vi "WLAN Rx Test Set WLAN INSTR RX.vi"(8 "error in (no error)":errorcluster, 10 "niDTS WLAN.lvlib:niDTS WLAN INSTR RX":refnum<class "niDTS WLAN INSTR RX.lvclass">, 11 "niDTS WLAN Rx Test in":refnum<class "niDTS WLAN Rx Test.lvclass">) -> (0 "error out":errorcluster, 3 "niDTS WLAN Rx Test out":refnum<class "niDTS WLAN Rx Test.lvclass">)   [LabVIEW 2015, in "niDTS WLAN.lvlib" / "niDTS WLAN Rx Test.lvclass"]
uses:
  niDTS WLAN Rx Test.lvclass
  Instrument/INSTR RX/niDTS WLAN INSTR RX.lvclass
  niDTS WLAN Rx Test.lvclass/niDTS WLAN Rx Test.ctl
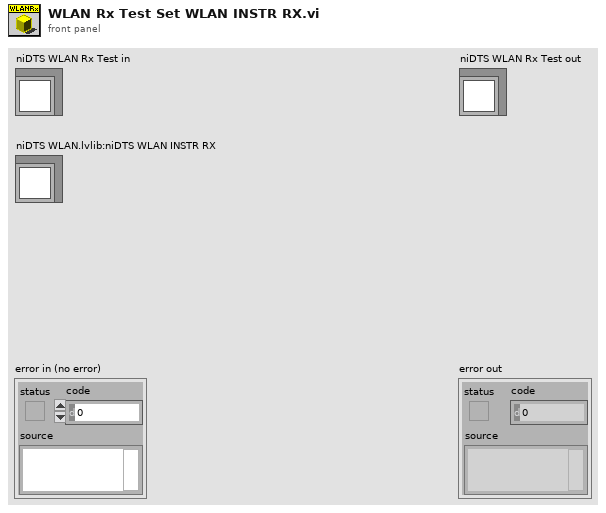
[diagram p1: front panel]
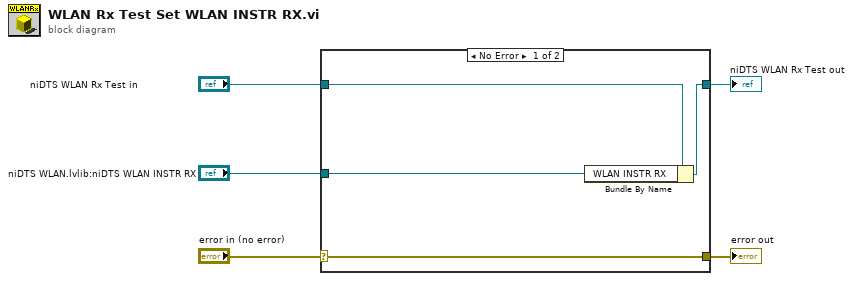
[diagram p0: block diagram]
diagram:
  n1 = case shown="No Error" "error in (no error)" {
    selector: "error in (no error)" -> [w9 w10]
    tunnel: [w9 w10] -> w4
    tunnel: [w7 w11] -> w2
    tunnel: "niDTS WLAN Rx Test in" -> [w8 w11]
    tunnel: "niDTS WLAN.lvlib:niDTS WLAN INSTR RX" -> [w6 _]
    frame No Error {
      n2 = Bundle By Name(cluster=w8, "WLAN INSTR RX"=w6) -> (w7:refnum<class "niDTS WLAN Rx Test.lvclass">)
    }
    frame Error {
    }
  }
  "error out" <- w4
  "niDTS WLAN Rx Test out" <- w2
